vi "Write Units.vi"(8 "error in (no error)":errorcluster, 10 "Units":T1, 11 "Level in":refnum<class "Level.lvclass">) -> (0 "error out":errorcluster, 3 "Level out":refnum<class "Level.lvclass">)   [LabVIEW 2020, in "Level.lvclass"]
uses:
  Level.lvclass
  LevelUnits.ctl
  Level.lvclass/Level.ctl
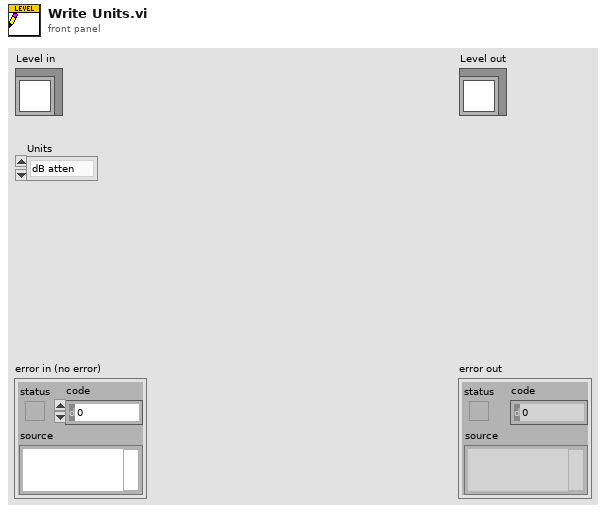
[diagram p1: front panel]
types:
  T1 = typedef "Level.lvclass/LevelUnits.ctl" = enum16{"dB atten", "dB SPL", "dB Vrms", "Volts", "dB mW", "mW", "dB HL", "dB SL"}
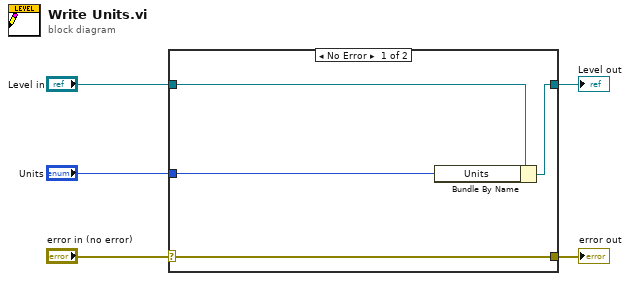
[diagram p0: block diagram]
diagram:
  n1 = case shown="No Error" "error in (no error)" {
    selector: "error in (no error)" -> [w9 w10]
    tunnel: [w9 w10] -> w4
    tunnel: [w7 w11] -> w2
    tunnel: "Level in" -> [w8 w11]
    tunnel: "Units" -> [w6 _]
    frame No Error {
      n2 = Bundle By Name(cluster=w8, "Units"=w6) -> (w7:refnum<class "Level.lvclass">)
    }
    frame Error {
    }
  }
  "error out" <- w4
  "Level out" <- w2
